vi "Alicat set 2.vi"(8 "error out 2":errorcluster, 10 "Byte array":u8[](array[numeric])=[65, 48, 48, 48, 48, 48, 13, 66, 48, 48, 48, 48, 48, 13, 67, 48, 48, 48, 48, 48, 13, 68, 48, 48, 48, 48, 48, 13, 69, 48, 48, 48, 48, 48, 13, 70, 48, 48, 48, 48, 48, 13, 71, 48, 48, 48, 48, 48, 13, 0, 0, 0, 0, 0, 0, 0, 0, 0, 0, 0, 0, 0, 0]) -> (0 "error out":errorcluster, 2 "MFC meas":i32[](array[numeric]))   [LabVIEW 2011]
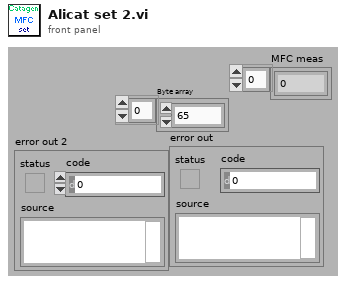
[diagram p1: front panel]
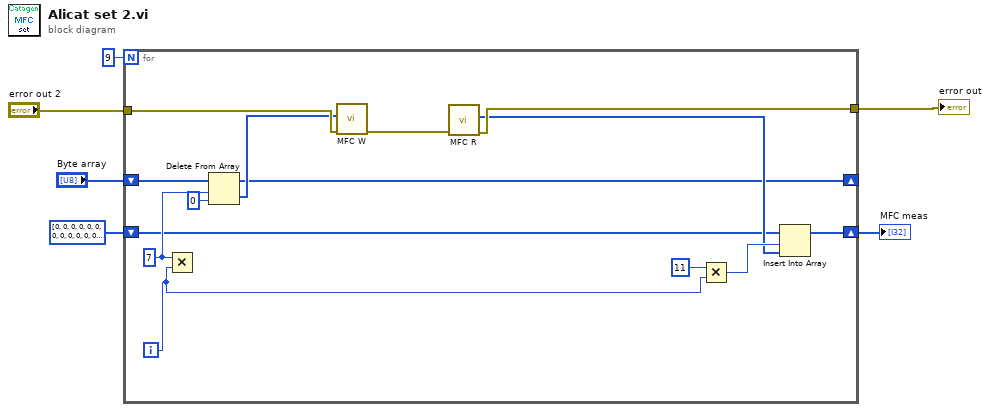
[diagram p0: block diagram]
diagram:
  n1 = for {
    N: 9 -> [_]
    tunnel: "error out 2" -> [w17]
    tunnel: [w15] -> w5
    shift-right: [w11] -> w3
    shift-left: i32[] [0, 0, 0, 0, 0, 0, 0, 0, 0, 0, 0, 0, 0, 0, 0, 0, 0, 0, 0, 0, 0, 0, 0, 0, 0, 0, 0, 0, 0, 0, 0, 0, 0, 0, 0, 0, 0, 0, 0, 0, 0, 0, 0, 0, 0, 0, 0, 0, 0, 0, 0, 0, 0, 0, 0, 0, 0, 0, 0, 0, 0, 0, 0, 0, 0, 0, 0, 0, 0, 0, 0, 0, 0, 0, 0, 0, 0, 0, 0, 0, 0, 0, 0, 0, 0, 0, 0, 0, 0, 0, 0, 0, 0, 0, 0, 0, 0, 0, 0] -> [w13]
    shift-right: [w7] -> _
    shift-left: "Byte array" -> [w8]
    i -> [w12]
    w20 = 7 ("x")
    n2 = Multiply(x=w20, y=w12) -> ()  [unwired: 1 out]
    n3 = Delete From Array(array=w8, length=w20, index=0) -> (deleted portion=w10:u8[], array with subset deleted=w7:u8[])
    n4 = call "MFC W.vi"("error out 2"=w17, "Byte array"=w10) -> ("error out"=w16:errorcluster)  [unwired: 9 in]
    n5 = call "MFC R.vi"("error in"=w16) -> ("Byte array"=w14:u8[], "error out"=w15:errorcluster)  [unwired: 8 in]
    n6 = Multiply(x=11, y=w12) -> (x*y=w18:i32)
    n7 = Insert Into Array(array=w13, index=w18, new element=w14) -> (w11:i32[])
  }
  "error out" <- w5
  "MFC meas" <- w3
